vi "Arduino_GetBoardListing.vi"() -> (2 "All Names":string[](array[string]))   [LabVIEW 2020]
panel:
  out "text":string
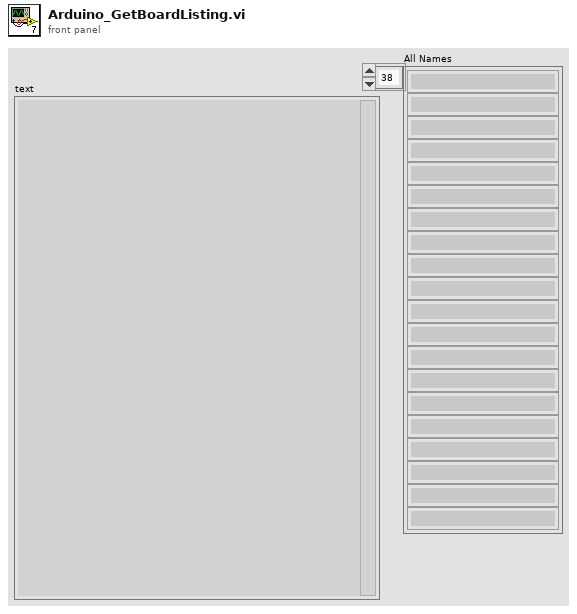
[diagram p1: front panel]
types:
  T1 = cluster{"packages":cluster{"name":string, "maintainer":string, "websiteURL":string, "platforms":cluster{"name":string, "architecture":string, "version":string, "category":string, "url":string, "archiveFileName":string, "checksum":string, "size":string, "boards":cluster{"name":string}[], "toolsDependencies":cluster{"packager":string, "name":string, "version":string}[]}[]}[]}
  T2 = cluster{"name":string, "maintainer":string, "websiteURL":string, "platforms":cluster{"name":string, "architecture":string, "version":string, "category":string, "url":string, "archiveFileName":string, "checksum":string, "size":string, "boards":cluster{"name":string}[], "toolsDependencies":cluster{"packager":string, "name":string, "version":string}[]}[]}[]
  T3 = cluster{"name":string, "architecture":string, "version":string, "category":string, "url":string, "archiveFileName":string, "checksum":string, "size":string, "boards":cluster{"name":string}[], "toolsDependencies":cluster{"packager":string, "name":string, "version":string}[]}[]
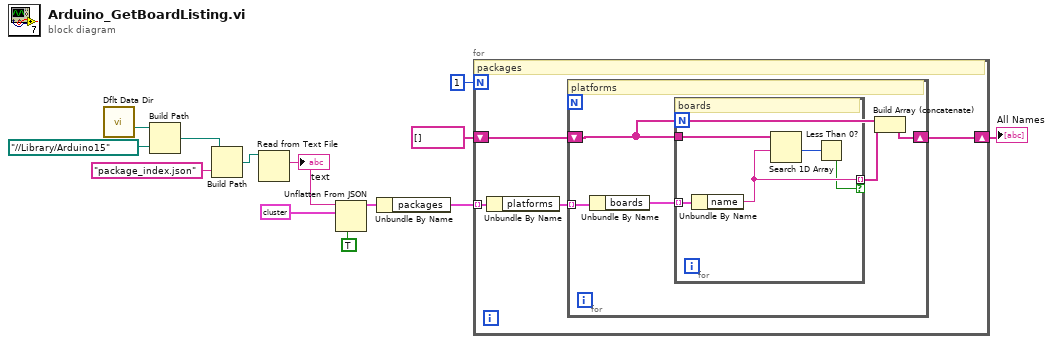
[diagram p0: block diagram]
diagram:
  n1 = call <vilib>:"Dflt Data Dir.vi"() -> ("App:Default Data Directory"=w13:path)
  n2 = Build Path(base path=w13, name or relative path=path "../../Library/Arduino15") -> (appended path=w5:path)
  n3 = Build Path(base path=w5, name or relative path="package_index.json") -> (appended path=w11:path)
  n4 = Read from Text File(file (use dialog)=w11) -> (text=w10:string)  [unwired: 3 in, 3 out]
  "text" <- w10
  n5 = Unflatten From JSON(JSON string=w10, type and defaults=T1 {"packages"=[{"name"="", "maintainer"="", "websiteURL"="", "platforms"=[{"name"=" ", "architecture"="", "version"="", "category"="", "url"="", "archiveFileName"="", "checksum"="", "size"="", "boards"=[{"name"=" "}], "toolsDependencies"=[{"packager"=" ", "name"="", "version"=""}]}]}]}, default null elements? (F)=TRUE) -> (value=w7:T1)  [unwired: 4 in, 1 out]
  n6 = Unbundle By Name(w7) -> ("packages"=w6:T2)
  n7 = for {
    N: 1 -> [_]
    tunnel: w6 -> [w16] mode=indexing
    shift-right: [w15] -> w4
    shift-left: string[] [] -> [w14]
    # "packages"
    n8 = Unbundle By Name(w16) -> ("platforms"=w17:T3)
    n9 = for {
      tunnel: w17 -> [w21] mode=indexing
      shift-right: [w18] -> w15
      shift-left: w14 -> [w20]
      # "platforms"
      n10 = Unbundle By Name(w21) -> ("boards"=w22:cluster{"name":string}[])
      n11 = for {
        tunnel: w22 -> [w27] mode=indexing
        tunnel: [w25] -> w19 mode=indexing if=w23
        tunnel: w20 -> [w26]
        # "boards"
        n12 = Unbundle By Name(w27) -> ("name"=w25:string)
        n13 = Search 1D Array(1D array=w26, element=w25) -> (index of element=w24:i32)  [unwired: 1 in]
        n14 = Less Than 0?(x=w24) -> (x < 0?=w23:bool)
      }
      n15 = Build Array (concatenate)(w20, w19) -> (w18:string[])
    }
  }
  "All Names" <- w4
